vi "Hardware_Reset.vi"(1 "Debug":bool) -> ()   [LabVIEW 2011]
doc: "This VI resets the MOCVD system by reinitializing all external hardware relays."
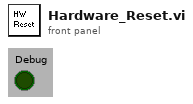
[diagram p1: front panel]
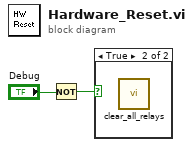
[diagram p0: block diagram]
diagram:
  n1 = Not(x="Debug") -> (.not. x?=w2:bool)
  n2 = case shown="True" w2 {
    frame False {
    }
    frame True {
      n3 = call "clear_all_relays.vi"() -> ()  [unwired: 2 out]
    }
  }
